vi "Init Data.vi"(8 "error in (no error)":errorcluster, 10 "Data Object":refnum<class "Factory Plugin Framework.lvclass">, 11 "QPA Measurement in":refnum<class "QPA Measurement.lvclass">) -> (0 "error out":errorcluster, 3 "QPA Measurement out":refnum<class "QPA Measurement.lvclass">)   [LabVIEW 2016, in "QPA Measurement.lvlib" / "QPA Measurement.lvclass"]
uses:
  QPA Measurement.lvclass
  Plugins/FPF.lvlibp/Factory Plugin Framework.lvclass
  QPA Measurement.lvclass/QPA Measurement.ctl
  Protected Methods/Read DC Pins.vi
  Protected Methods/Read PAE Pins.vi
  Protected Methods/Read RF Waveform Database.vi
  Protected Methods/Read Default Steps Database.vi
  Protected Methods/Read Dut Setup Step.vi
  Protected Methods/Read DUT Setup Parameters.vi
  Protected Methods/Read External Network Step.vi
  Protected Methods/Read Sequence Reference.vi
  Protected Methods/Read Measurement Name.vi
  Protected Methods/Read External Network Present.vi
  Protected Methods/Read TSF MNGR.vi
  Protected Methods/Read Test Group Manager.vi
  Protected Methods/Write DC Pins.vi
  Protected Methods/Write PAE Pins.vi
  Protected Methods/Write RF Waveform Database.vi
  Protected Methods/Write Default Steps Database.vi
  Protected Methods/Write Dut Setup Step.vi
  Protected Methods/Write DUT Setup Parameters.vi
  Protected Methods/Write External Network Step.vi
  Protected Methods/Write Sequence Reference.vi
  Protected Methods/Write Measurement Name.vi
  Protected Methods/Write External Network Present.vi
  Protected Methods/Write TSF MNGR.vi
  Protected Methods/Write Test Group Manager.vi
  Plugins/Measurement Interface.lvlibp/Measurement Interface.lvclass
  Waveform Manager/QPA MSMT Waveform Manager.lvclass
  Plugins/TSF Parser.lvlibp/TSF Parser.lvclass
  Plugins/Test Group Manager.lvlibp/Test Group Manager.lvclass
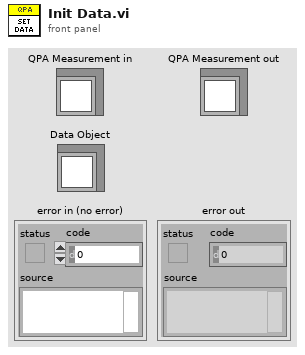
[diagram p1: front panel]
types:
  T1 = typedef "QPA Measurement.lvlib/QPA Measurement.lvclass/Parameter.ctl" = cluster{"Name":string, "PropertyObject Type":enum16{"Container", "String", "Boolean", "Number", "NamedType", "Reference", "Array", "Aperture Time"}}
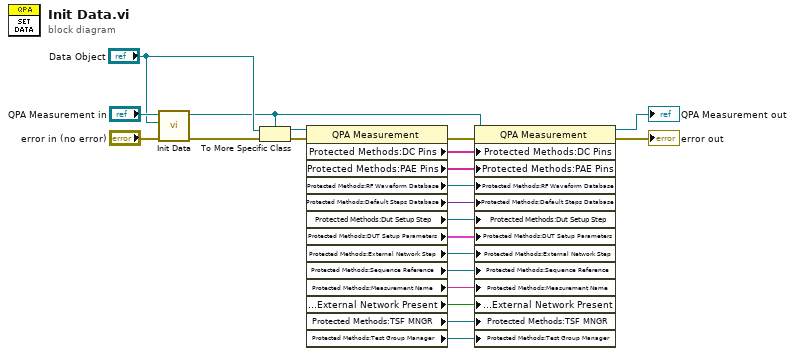
[diagram p0: block diagram]
diagram:
  n1 = call-parent "Init Data.vi"("error in (no error)"="error in (no error)", "Data Object"="Data Object", "Measurement Interface in"="QPA Measurement in") -> ("error out"=w22:errorcluster, "Measurement Interface out"=w16:refnum<class "QPA Measurement.lvclass">)  [unwired: 7 in]
  n2 = To More Specific Class(target class=w16, reference="Data Object", error in=w22) -> (specific class reference=w17:refnum<class "QPA Measurement.lvclass">, error out=w19:errorcluster)
  n3 = property class="QPA Measurement"(reference=w17, error in=w19) -> (error out=w13:errorcluster, "Protected Methods:DC Pins"=w12:string[], "Protected Methods:PAE Pins"=w11:string[], "Protected Methods:RF Waveform Database"=w10:refnum<class "QPA MSMT Waveform Manager.lvclass">, "Protected Methods:Default Steps Database"=w9:variant, "Protected Methods:Dut Setup Step"=w8:refnum<k7>, "Protected Methods:DUT Setup Parameters"=w7:T1[], "Protected Methods:External Network Step"=w6:refnum<k7>, "Protected Methods:Sequence Reference"=w5:refnum<k7>, "Protected Methods:Measurement Name"=w4:string, "Protected Methods:External Network Present"=w3:bool, "Protected Methods:TSF MNGR"=w2:refnum<class "TSF Parser.lvclass">, "Protected Methods:Test Group Manager"=w1:refnum<data-value>)  [unwired: 1 out]
  n4 = property class="QPA Measurement"(reference=w16, error in=w13, "Protected Methods:DC Pins"=w12, "Protected Methods:PAE Pins"=w11, "Protected Methods:RF Waveform Database"=w10, "Protected Methods:Default Steps Database"=w9, "Protected Methods:Dut Setup Step"=w8, "Protected Methods:DUT Setup Parameters"=w7, "Protected Methods:External Network Step"=w6, "Protected Methods:Sequence Reference"=w5, "Protected Methods:Measurement Name"=w4, "Protected Methods:External Network Present"=w3, "Protected Methods:TSF MNGR"=w2, "Protected Methods:Test Group Manager"=w1) -> (reference out=→"QPA Measurement out":refnum<class "QPA Measurement.lvclass">, error out=→"error out":errorcluster)
